vi "disarm.vi"(1 "error in":errorcluster, 2 "address string":string="24") -> (0 "error out":errorcluster)   [LabVIEW 2012]
panel:
  # "Disarm Measurement Mode 6221"
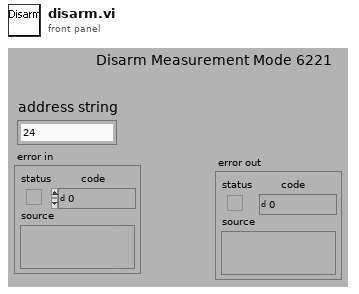
[diagram p1: front panel]
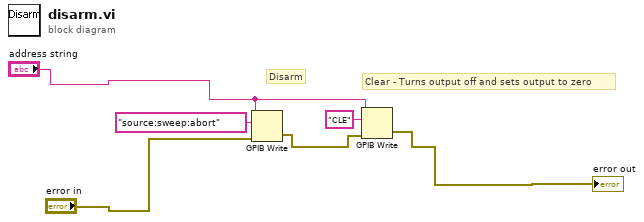
[diagram p0: block diagram]
diagram:
  # "Clear - Turns output off and sets output to zero"
  # "Disarm"
  n1 = GPIB Write(0:"address string", 1:"source:sweep:abort" ("data"), 3:"error in") -> (6:w2:errorcluster)  [unwired: 2 in, 1 out]
  n2 = GPIB Write(0:"address string", 1:"CLE" ("data"), 3:w2) -> (6:→"error out":errorcluster)  [unwired: 2 in, 1 out]
